vi "SetLogFormatter.vi"(8 "Error in (no error)":errorcluster, 10 "LogFormatterInterface in":refnum<class "LogFormatterInterface.lvclass">, 11 "LogWriterEmail in":refnum<class "LogWriterEmail.lvclass">) -> (0 "Error out":errorcluster, 3 "LogWriterEmail out":refnum<class "LogWriterEmail.lvclass">)   [LabVIEW 2011, in "LogWriterEmail.lvclass"]
uses:
  LogWriterEmail.lvclass
  Formatter/LogFormatterInterface/LogFormatterInterface.lvclass
  LogWriterInterface/LogWriterInterface.lvclass
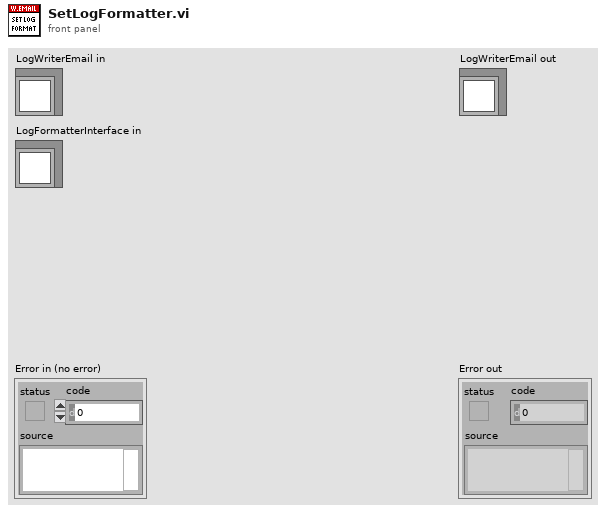
[diagram p1: front panel]
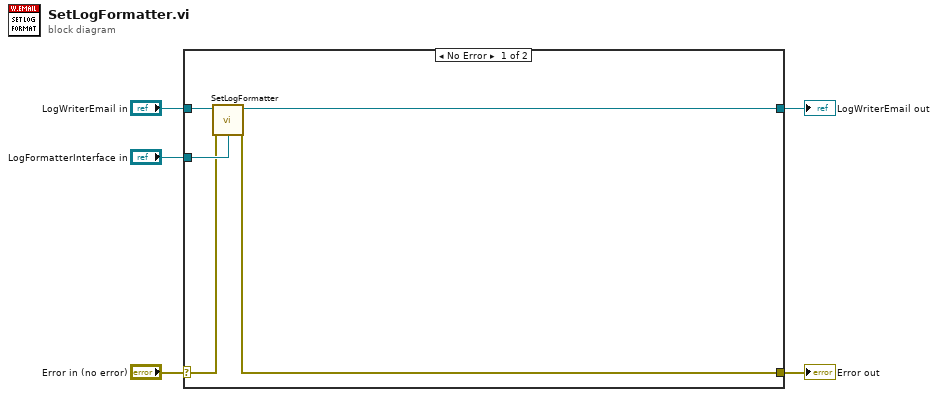
[diagram p0: block diagram]
diagram:
  n1 = case shown="No Error" "Error in (no error)" {
    selector: "Error in (no error)" -> [w7 w12]
    tunnel: [w6 w12] -> w4
    tunnel: [w10 w11] -> w2
    tunnel: "LogWriterEmail in" -> [w8 w11]
    tunnel: "LogFormatterInterface in" -> [w9 _]
    frame No Error {
      n2 = call-parent "SetLogFormatter.vi"("Error in (no error)"=w7, "LogFormatterInterface in"=w9, "LogWriterInterface in"=w8) -> ("Error out"=w6:errorcluster, "LogWriterInterface out"=w10:refnum<class "LogWriterEmail.lvclass">)  [unwired: 7 in]
    }
    frame Error {
    }
  }
  "Error out" <- w4
  "LogWriterEmail out" <- w2
